vi "spilib_setopts.vi"(6 "clk_idle_high":bool=TRUE, 8 "error in (no error)":errorcluster, 9 "sample_on_trailing":bool=TRUE, 10 "msb_first":bool=TRUE, 11 "handle":i32) -> (0 "error out":errorcluster, 3 "handle out":i32)   [LabVIEW 2017]
uses:
  <vilib>/Utility/error.llb/Error Cluster From Error Code.vi
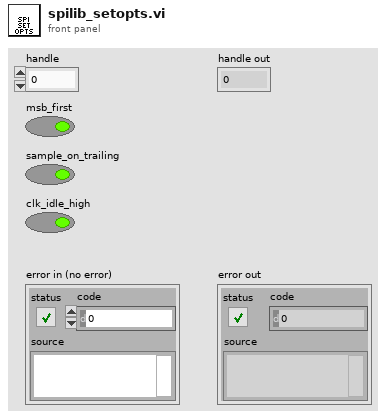
[diagram p1: front panel]
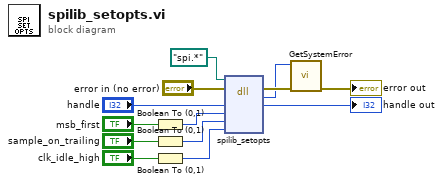
[diagram p0: block diagram]
diagram:
  n1 = Boolean To (0,1)(Boolean="msb_first") -> (0, 1=w3:i16)
  n2 = Boolean To (0,1)(Boolean="sample_on_trailing") -> (0, 1=w2:i16)
  n3 = Boolean To (0,1)(Boolean="clk_idle_high") -> (0, 1=w1:i16)
  n4 = dll-call lib="?" fn="spilib_setopts"(path in=path "spi.*", error in="error in (no error)", "handle"="handle", "msb_first"=w3, "sample_on_trailing"=w2, "clk_idle_high"=w1) -> (error out=w12:errorcluster, "return type"=w10:i32, "handle"=→"handle out":i32)  [unwired: 4 in, 1 out]
  n5 = call <vilib>:"GetSystemError.vi"("error in (no error)"=w12, "Retval"=w10) -> ("error out"=→"error out":errorcluster)  [unwired: 9 in]
